vi "Configure S3DK.vi"(8 "error in (no error)":errorcluster, 11 "Settings IN":T1={"State"=enum."Idle", "Settings"="", "Online"=FALSE, "S3DK"={"Signals"={"Phasor"=[], "Analog"=[], "Digital"=[]}}, "CSV"={"Index"=0, "Parcel Length"=0, "EOF?"=FALSE, "Config"={"Mode"=enum."Full timestamp", "delimiter (\\t)"="\t", "Path"=path "", "Rectangular?"=FALSE}}}) -> (0 "error out":errorcluster, 3 "Settings OUT":T1={"State"=enum."Idle", "Settings"="", "Online"=FALSE, "S3DK"={"Signals"={"Phasor"=[], "Analog"=[], "Digital"=[]}}, "CSV"={"Index"=0, "Parcel Length"=0, "EOF?"=FALSE, "Config"={"Mode"=enum."Full timestamp", "delimiter (\\t)"="\t", "Path"=path "", "Rectangular?"=FALSE}}})   [LabVIEW 2017, in "Acquisition.lvlib"]
doc: "Configure the hardware."
uses:
  Acquisition.lvlib
  Acquisition Settings.ctl
  Acquisition State.ctl
  support/libs/CSV Reader/Mode CSV reader.ctl
  <vilib>/S3DK/PMU Recorder Light/PMU Recorder Light.lvlib
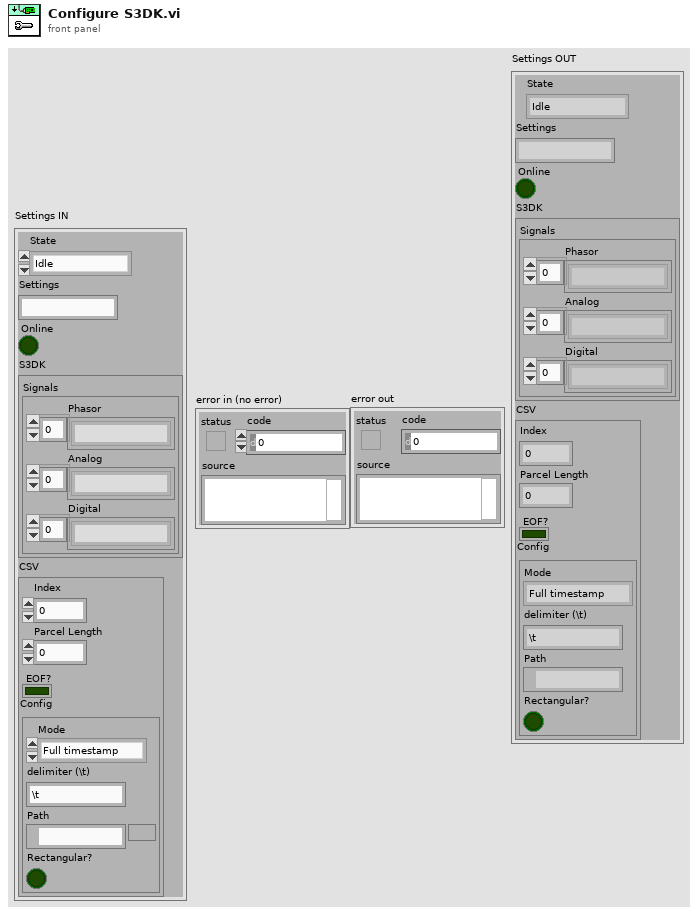
[diagram p1: front panel]
types:
  T1 = typedef "Acquisition.lvlib/Acquisition Settings.ctl" = cluster{"State":T2, "Settings":string, "Online":bool, "S3DK":cluster{"Signals":cluster{"Phasor":string[], "Analog":string[], "Digital":string[]}}, "CSV":cluster{"Index":i32, "Parcel Length":i32, "EOF?":bool, "Config":cluster{"Mode":T3, "delimiter (\\t)":string, "Path":path, "Rectangular?":bool}}}
  T2 = typedef "Acquisition.lvlib/Acquisition State.ctl" = enum16{"Idle", "Idle S3DK", "Acquiring S3DK", "Idle CSV", "Acquiring CSV"}
  T3 = typedef "Mode CSV reader.ctl" = enum16{"Full timestamp", "Relative Time", "Seconds Time", "Nanoseconds Time"}
  T4 = enum16{"Filter Signals", "Get All Signal Names", "Select Signals on Name", "Select Frequency Only", "Get Selected Signal Names"}
  T5 = cluster{"Phasor":string[], "Analog":string[], "Digital":string[]}
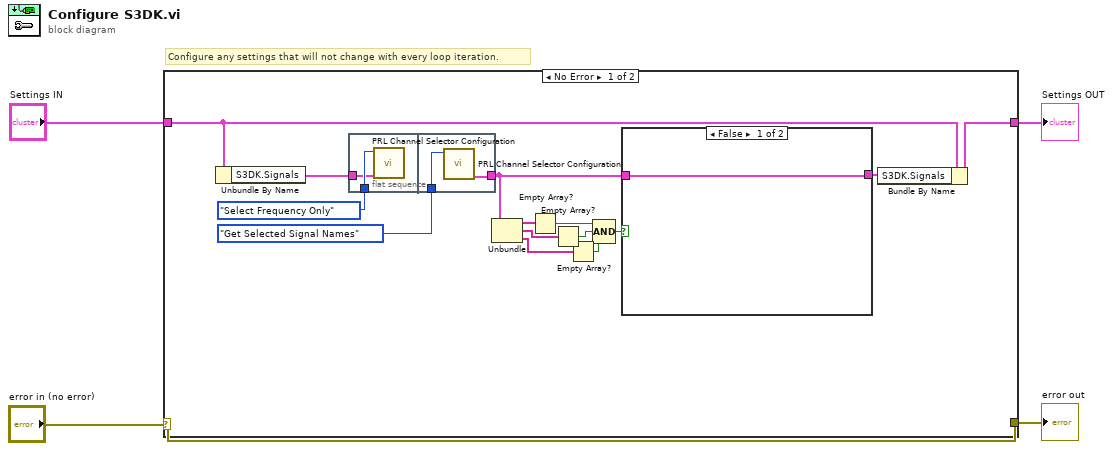
[diagram p0: block diagram]
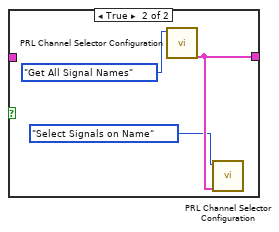
[diagram p2: hidden frame]
diagram:
  # "Configure any settings that will not change with every loop iteration."
  n1 = case shown="No Error" "error in (no error)" {
    selector: "error in (no error)" -> [w19 w28]
    tunnel: [w19 w28] -> w3
    tunnel: "Settings IN" -> [w16 w29]
    tunnel: [w15 w29] -> w1
    frame No Error {
      n2 = Unbundle By Name(w16) -> ("S3DK.Signals"=w14:T5)
      n3 = flat-sequence {
        tunnel: T4."Select Frequency Only" ("Action") -> [w25]
        tunnel: w14 -> [w24]
        tunnel: [w27] -> w6
        tunnel: T4."Get Selected Signal Names" ("Action") -> [w26]
        frame #0 {
          n4 = call <vilib>:"PRL Channel Selector Configuration.vi"("Signal Names In"=w24, "Action"=w25) -> ()  [unwired: 9 in, 1 out]
        }
        frame #1 {
          n5 = call <vilib>:"PRL Channel Selector Configuration.vi"("Action"=w26) -> ("Signal Names Out"=w27:T5)  [unwired: 10 in]
        }
      }
      n6 = Unbundle(w6) -> ("Phasor"=w13:string[], "Analog"=w12:string[], "Digital"=w11:string[])
      n7 = Empty Array?(array=w13) -> (empty?=w10:bool)
      n8 = Empty Array?(array=w12) -> (empty?=w9:bool)
      n9 = Empty Array?(array=w11) -> (empty?=w8:bool)
      n10 = Compound Arithmetic op=AND(w10, w9, w8) -> (w7:bool)
      n11 = case shown="False" w7 {
        tunnel: [w20 w22] -> w5
        tunnel: w6 -> [w20 _]
        frame False {
        }
        frame True {
          n12 = call <vilib>:"PRL Channel Selector Configuration.vi"("Action"=T4."Get All Signal Names") -> ("Signal Names Out"=w22:T5)  [unwired: 10 in]
          n13 = call <vilib>:"PRL Channel Selector Configuration.vi"("Signal Names In"=w22, "Action"=T4."Select Signals on Name") -> ()  [unwired: 9 in, 1 out]
        }
      }
      n14 = Bundle By Name(cluster=w16, "S3DK.Signals"=w5) -> (w15:T1)
    }
    frame Error {
    }
  }
  "Settings OUT" <- w1
  "error out" <- w3
